vi "Scan_Image.vi"(0 "array":i32[][](array[numeric]), 11 "error in (no error)":errorcluster) -> (3 "Image":T1(plugin-control), 15 "error out":errorcluster)   [LabVIEW 2011]
uses:
  Variables/GlobalSetGetPixelOfRoi.vi
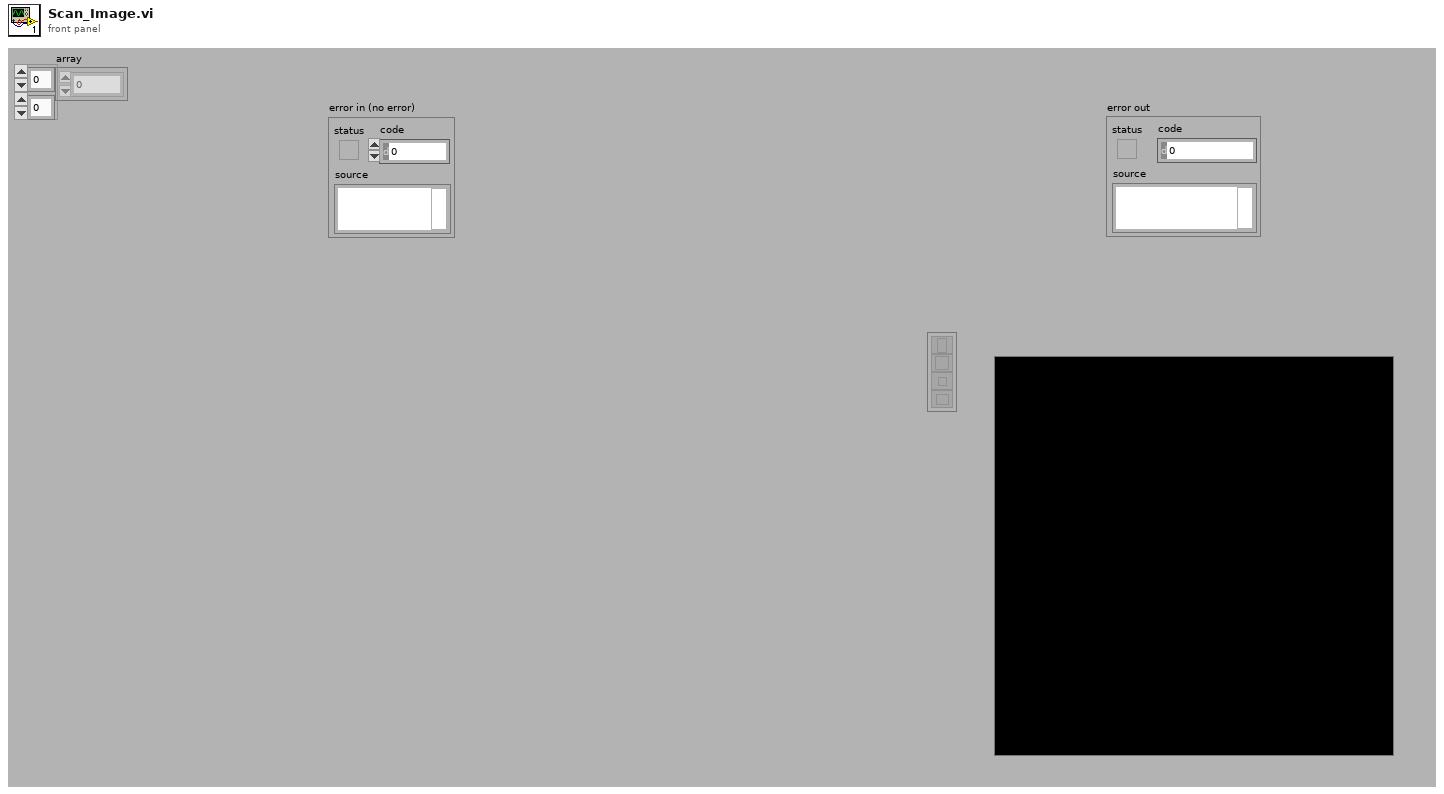
[diagram p1: front panel]
types:
  T1 = typedef "IMAQ Image.ctl" = refnum<image>
  T2 = cluster{"Left":i32, "Top":i32, "Right":i32, "Bottom":i32}
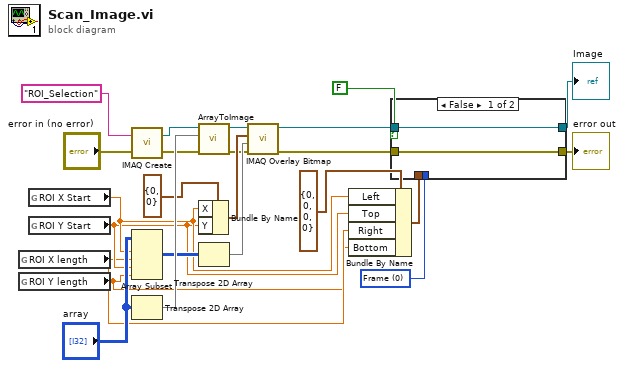
[diagram p0: block diagram]
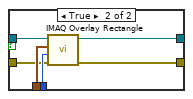
[diagram p2: hidden frame]
diagram:
  w18 = u32 0 items=["Frame", "Fill", "Highlight"] ("Drawing Mode (Frame)")
  n1 = global read "GlobalSetGetPixelOfRoi.vi" "ROI X length"() -> (w3:dbl)
  n2 = global read "GlobalSetGetPixelOfRoi.vi" "ROI Y length"() -> (w2:dbl)
  n3 = global read "GlobalSetGetPixelOfRoi.vi" "ROI X Start"() -> (w5:dbl)
  n4 = global read "GlobalSetGetPixelOfRoi.vi" "ROI Y Start"() -> (w4:dbl)
  n5 = call "IMAQ Create"("Image Name"="ROI_Selection", "error in (no error)"="error in (no error)") -> ("New Image"=w24:T1, "error out"=w22:errorcluster)  [unwired: 3 in]
  n6 = Array Subset(array="array", index (row)=w5, length (row)=w3, index (col)=w4, length (col)=w2) -> (w6:i32[][])
  n7 = Transpose 2D Array(2D array="array") -> (transposed array=w23:i32[][])
  n8 = call "ArrayToImage.vi"("error in (no error)"=w22, "Image Pixels (U8)"=w23, "Image"=w24) -> ("error out"=w7:errorcluster, "Image Out"=w20:T1)  [unwired: 7 in]
  n9 = Bundle By Name(cluster=cluster{"X":i32, "Y":i32} {"X"=0, "Y"=0} ("Top Left Point"), "X"=w5, "Y"=w4) -> (w13:cluster{"X":i32, "Y":i32})
  n10 = Transpose 2D Array(2D array=w6) -> (transposed array=w12:i32[][])
  n11 = call "IMAQ Overlay Bitmap"("error in (no error)"=w7, "Bitmap"=w12, "Top Left Point"=w13, "Image"=w20) -> ("error out"=w15:errorcluster, "Image Out"=w16:T1)  [unwired: 6 in]
  n12 = Bundle By Name(cluster=T2 {"Left"=0, "Top"=0, "Right"=0, "Bottom"=0} ("Rectangle"), "Left"=w5, "Top"=w4, "Right"=w3, "Bottom"=w2) -> (w17:T2)
  n13 = case shown="False" FALSE ("Boolean") {
    tunnel: w18 -> [_ w32]
    tunnel: w17 -> [_ w31]
    tunnel: w16 -> [w26 w30]
    tunnel: w15 -> [w25 w29]
    tunnel: [w26 w28] -> w11
    tunnel: [w25 w27] -> w9
    frame False {
    }
    frame True {
      n14 = call "IMAQ Overlay Rectangle"("error in (no error)"=w29, "Drawing Mode (Frame)"=w32, "Rectangle"=w31, "Image"=w30) -> ("error out"=w27:errorcluster, "Image Out"=w28:T1)  [unwired: 6 in]
    }
  }
  "Image" <- w11
  "error out" <- w9
